vi "Write Index.vi"(8 "error in (no error)":errorcluster, 10 "Index":i32, 11 "Local Bus_Access in":refnum<class "Local Bus_U8.lvclass">) -> (0 "error out":errorcluster, 3 "Local Bus_Access out":refnum<class "Local Bus_U8.lvclass">)   [LabVIEW 2021, in "Local Bus_U8.lvclass"]
uses:
  Local Bus_U8.lvclass
  Local Bus_U8.lvclass/Local Bus_U8.ctl
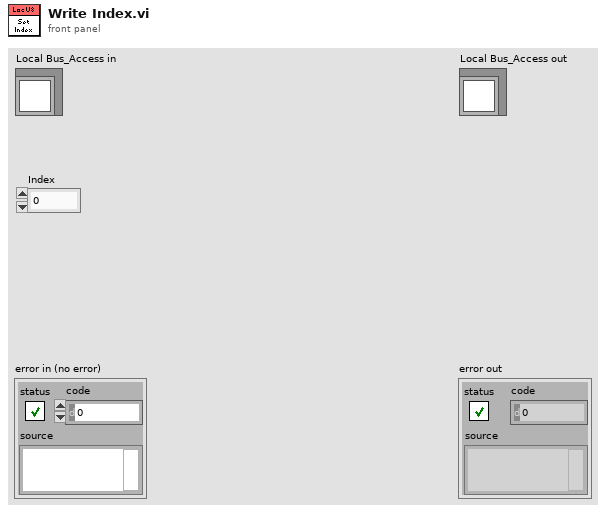
[diagram p1: front panel]
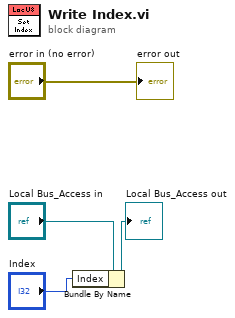
[diagram p0: block diagram]
diagram:
  n1 = Bundle By Name(cluster="Local Bus_Access in", "Index"="Index") -> (→"Local Bus_Access out":refnum<class "Local Bus_U8.lvclass">)
  "error out" <- "error in (no error)"
